vi "uPython_Initialize.vi"(11 "VISA Refnum in":refnum<visa-resource-name>) -> (0 "error out":errorcluster, 3 "VISA Refnum out":refnum<visa-resource-name>)   [LabVIEW 2016]
uses:
  <vilib>/Instr/_visa.llb/VISA Configure Serial Port (Instr).vi
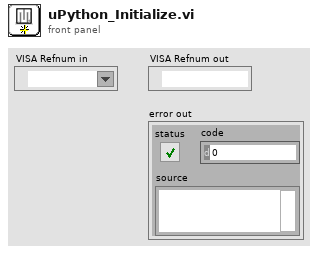
[diagram p1: front panel]
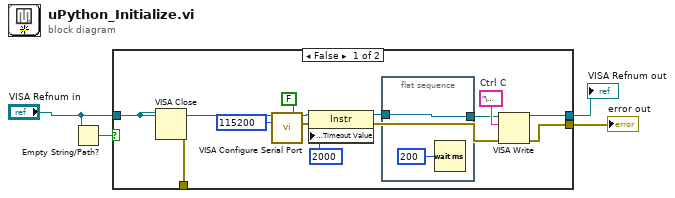
[diagram p0: block diagram]
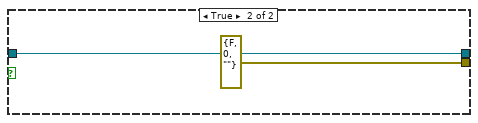
[diagram p2: hidden frame]
diagram:
  n1 = Empty String/Path?(string/path="VISA Refnum in") -> (empty?=w4:bool)
  n2 = case shown="False" w4 {
    tunnel: [w12 w21] -> w1
    tunnel: [w9 errorcluster {"status"=FALSE, "code"=0, "source"=""} ("error out")] -> w2
    tunnel: "VISA Refnum in" -> [w5 w21]
    tunnel: [w6 _] -> _
    frame False {
      w11 = "\u0003"  # Ctrl C
      n3 = VISA Close(VISA resource name=w5) -> (error out=w6:errorcluster)  [unwired: 1 in]
      n4 = call-poly "VISA Configure Serial Port"("VISA resource name"=w5, "Enable Termination\nChar (T)"=FALSE ("Enable Termination\nChar (T)"), "baud rate (9600)"=u32 115200) -> ("VISA resource name out"=w17:refnum<visa-resource-name>, "error out"=w14:errorcluster)  [unwired: 11 in]
      n5 = property class="Instr"(reference=w17, error in=w14, "General Settings:Timeout Value"=u32 2000) -> (reference out=w7:refnum<visa-resource-name>, error out=w10:errorcluster)
      n6 = flat-sequence {
        tunnel: [w18] -> w8
        tunnel: w7 -> [w18]
        frame #0 {
          n7 = Wait (ms)(milliseconds to wait=u32 200) -> ()  [unwired: 1 out]
        }
      }
      n8 = VISA Write(VISA resource name=w8, write buffer=w11, error in (no error)=w10) -> (VISA resource name out=w12:refnum<visa-resource-name>, error out=w9:errorcluster)  [unwired: 1 out]
    }
    frame True {
    }
  }
  "error out" <- w2
  "VISA Refnum out" <- w1
